vi "Benchmark SV Receive LV2012 - NI Verified.vi"() -> ()   [LabVIEW 2015]
panel:
  out "data out":dbl
  in  "stop":bool
  # "Overview:  Coding that exemplifies how to benchmark the communication of Shared Variables.\nRequirements: LabVIEW 2012 or compatible\nInstructions:\n1. Run this VI\n2. Watch the amount of time it takes to communicate on the \"Benchmark SV Send  LV2012 - NI Verified.vi\" \n3. Stop both VIs"
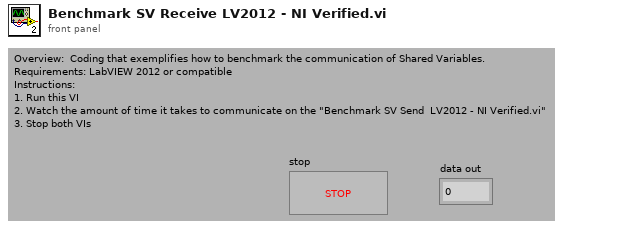
[diagram p1: front panel]
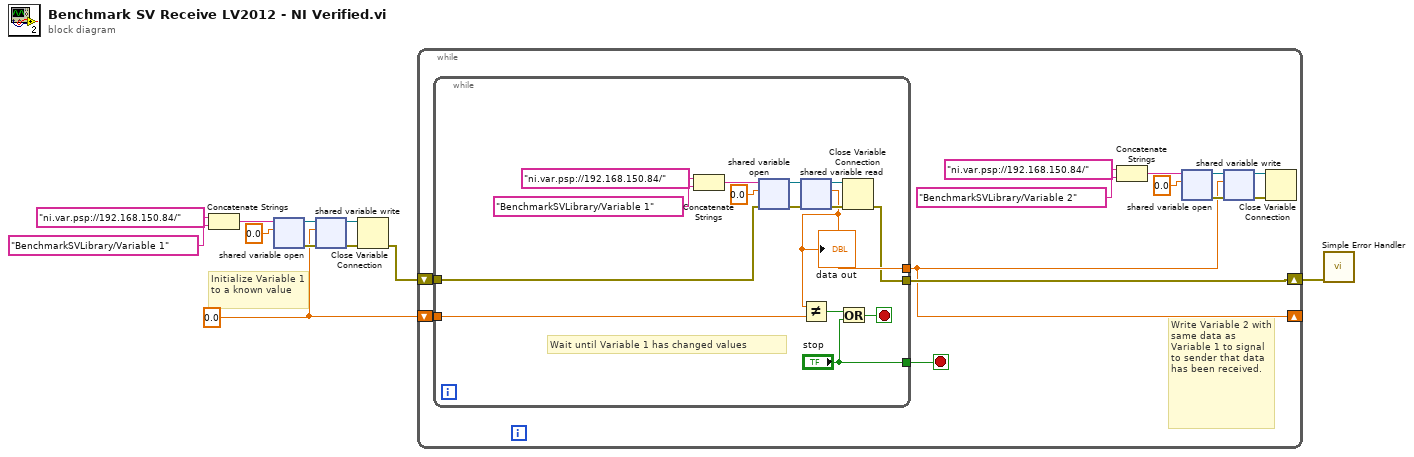
[diagram p0: block diagram]
diagram:
  w2 = 0.0 ("Variable 1")
  # "Initialize Variable 1 to a known value"
  n1 = Concatenate Strings("ni.var.psp://192.168.150.84/" ("string"), "BenchmarkSVLibrary/Variable 1") -> (w10:string)
  n2 = shared-variable-open(w10, 0.0 ("Variable 1")) -> (w7:refnum<k21>, w5:errorcluster)  [unwired: 2 in]
  n3 = shared-variable-write(w7, w5, w2) -> (w6:refnum<k21>, w4:errorcluster)
  n4 = Close Variable Connection(8:w4, 11:w6) -> (0:w1:errorcluster)
  n5 = while {
    shift-right: [w12] -> _
    shift-left: w2 -> [w24]
    shift-right: [w21] -> w11
    shift-left: w1 -> [w22]
    stop <- w23 stop-if-true
    # "Write Variable 2 with same data as Variable 1 to signal to sender that data has been received."
    n6 = while {
      tunnel: w24 -> [w39]
      tunnel: [w27] -> w12
      tunnel: ["stop"] -> w23
      tunnel: [w26] -> w21
      tunnel: w22 -> [w25]
      stop <- w36 stop-if-true
      # "Wait until Variable 1 has changed values"
      n7 = Concatenate Strings("ni.var.psp://192.168.150.84/" ("string"), "BenchmarkSVLibrary/Variable 1") -> (w33:string)
      n8 = shared-variable-open(w33, w25, 0.0 ("Variable 1")) -> (w32:refnum<k21>, w31:errorcluster)  [unwired: 1 in]
      n9 = shared-variable-read(w32, w31) -> (w30:refnum<k21>, w29:errorcluster, w27:dbl)  [unwired: 1 out]
      "data out" <- w27
      n10 = Not Equal?(x=w27, y=w39) -> (x != y?=w38:bool)
      n11 = Or(x=w38, y="stop") -> (x .or. y?=w36:bool)
      n12 = Close Variable Connection(8:w29, 11:w30) -> (0:w26:errorcluster)
    }
    n13 = Concatenate Strings("ni.var.psp://192.168.150.84/" ("string"), "BenchmarkSVLibrary/Variable 2") -> (w18:string)
    n14 = shared-variable-open(w18, 0.0 ("Variable 1")) -> (w17:refnum<k21>, w16:errorcluster)  [unwired: 2 in]
    n15 = shared-variable-write(w17, w16, w12) -> (w15:refnum<k21>, w14:errorcluster)
    n16 = Close Variable Connection(8:w14, 11:w15) -> ()  [unwired: 1 out]
  }
  n17 = call <vilib>:"Simple Error Handler.vi"("error in (no error)"=w11) -> ()  [unwired: 4 in, 5 out]
